vi "Select.vi"() -> ()   [LabVIEW 2019]
panel:
  in  "Flag":bool
  out "Output 2":string
  out "Output":string
  in  "a":dbl
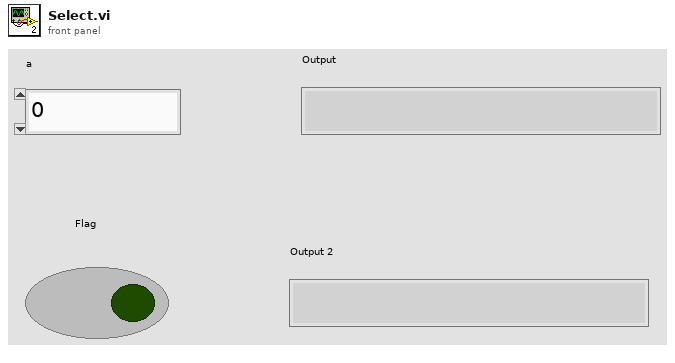
[diagram p1: front panel]
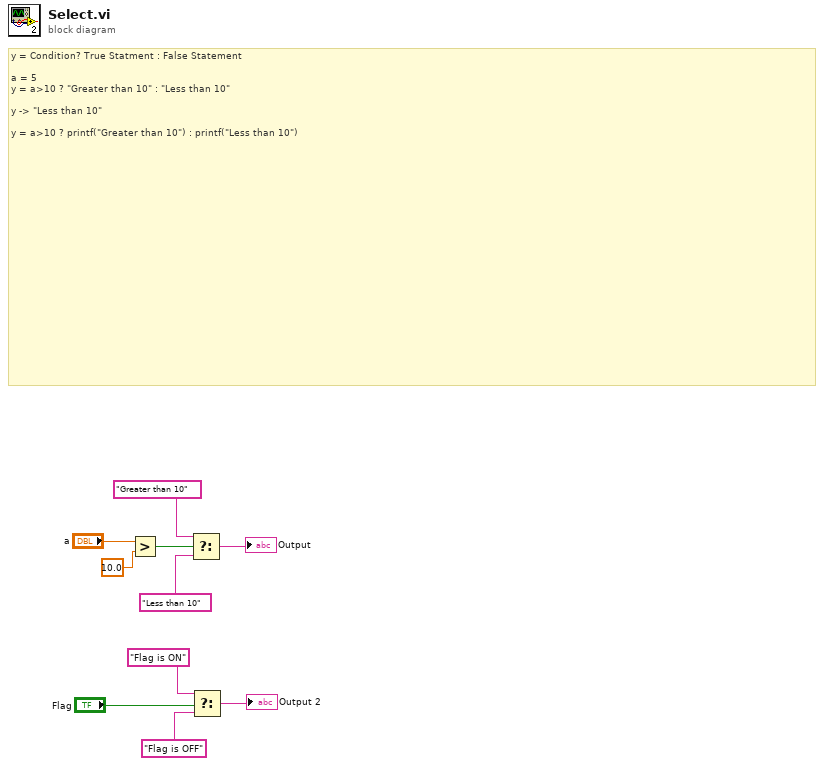
[diagram p0: block diagram]
diagram:
  # "y = Condition? True Statment : False Statement\n\na = 5\ny = a>10 ? \"Greater than 10\" : \"Less than 10\"\n\ny -> \"Less than 10\"\n\ny = a>10 ? printf(\"Greater than 10\") : printf(\"Less than 10\")"
  n1 = Greater?(x="a", y=10.0) -> (0:w8:bool)
  n2 = Select(t="Greater than 10", s=w8, f="Less than 10") -> (s? t:f=→"Output":string)
  n3 = Select(t="Flag is ON", s="Flag", f="Flag is OFF") -> (s? t:f=→"Output 2":string)
